vi "PickBall.vi"() -> ()   [LabVIEW 2017]
panel:
  out "Servo Position  2":u8
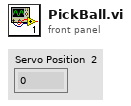
[diagram p1: front panel]
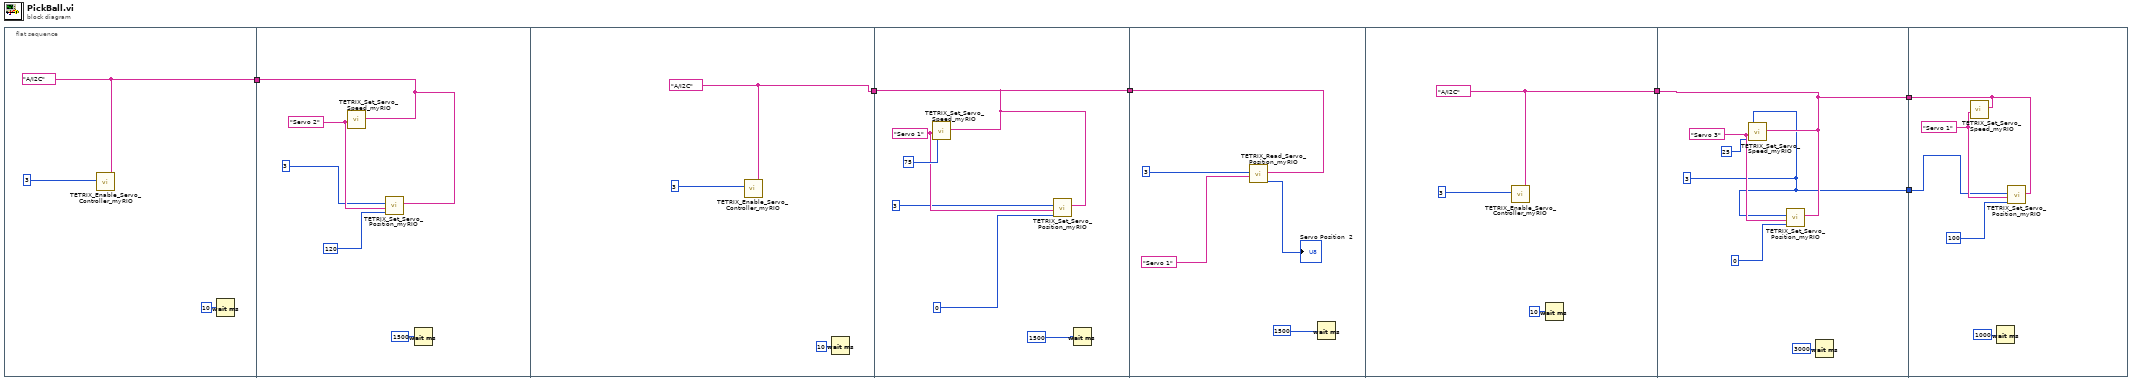
[diagram p0: block diagram]
diagram:
  n1 = flat-sequence {
    tunnel: [w8] -> w5
    tunnel: w5 -> [w10]
    tunnel: [w15] -> w3
    tunnel: [w18] -> w6
    tunnel: w3 -> [w18]
    tunnel: w6 -> [w27]
    tunnel: [w30] -> w4
    tunnel: w4 -> [w34]
    tunnel: [w33] -> w2
    tunnel: [w34] -> w1
    tunnel: w2 -> [w39]
    tunnel: w1 -> [w38]
    frame #0 {
      w8 = tag "A/I2C" ("myRIO MXP Port A/B")
      n2 = call <vilib>:"TETRIX_Enable_Servo_Controller_myRIO.vi"("myRIO MXP Port A/B"=w8, "Controller ID#  (I2C Address)"=u8 3) -> ()  [unwired: 5 in, 1 out]
      n3 = Wait (ms)(milliseconds to wait=u32 10) -> ()  [unwired: 1 out]
    }
    frame #1 {
      w14 = "Servo 2" ("Select Channel")
      n4 = call <vilib>:"TETRIX_Set_Servo_Speed_myRIO.vi"("myRIO MXP Port A/B"=w10, "Select Channel"=w14) -> ()  [unwired: 5 in, 1 out]
      n5 = call <vilib>:"TETRIX_Set_Servo_Position_myRIO.vi"("myRIO MXP Port A/B"=w10, "Set Servo Position (0 - 180 degrees)"=u8 120, "Select Channel"=w14, "Controller ID#  (I2C Address)"=u8 3) -> ()  [unwired: 3 in, 1 out]
      n6 = Wait (ms)(milliseconds to wait=u32 1500) -> ()  [unwired: 1 out]
    }
    frame #2 {
      w15 = tag "A/I2C" ("myRIO MXP Port A/B")
      n7 = call <vilib>:"TETRIX_Enable_Servo_Controller_myRIO.vi"("myRIO MXP Port A/B"=w15, "Controller ID#  (I2C Address)"=u8 3) -> ()  [unwired: 5 in, 1 out]
      n8 = Wait (ms)(milliseconds to wait=u32 10) -> ()  [unwired: 1 out]
    }
    frame #3 {
      w22 = "Servo 1" ("Select Channel")
      n9 = call <vilib>:"TETRIX_Set_Servo_Speed_myRIO.vi"("myRIO MXP Port A/B"=w18, "Set Servo Speed (0 - 100 percent)"=u8 75, "Select Channel"=w22) -> ()  [unwired: 4 in, 1 out]
      n10 = call <vilib>:"TETRIX_Set_Servo_Position_myRIO.vi"("myRIO MXP Port A/B"=w18, "Set Servo Position (0 - 180 degrees)"=u8 0, "Select Channel"=w22, "Controller ID#  (I2C Address)"=u8 3) -> ()  [unwired: 3 in, 1 out]
      n11 = Wait (ms)(milliseconds to wait=u32 1500 ("millisecond timer value")) -> ()  [unwired: 1 out]
    }
    frame #4 {
      n12 = call <vilib>:"TETRIX_Read_Servo_Position_myRIO.vi"("myRIO MXP Port A/B"=w27, "Select Channel"="Servo 1", "Controller ID#  (I2C Address)"=u8 3) -> ("Servo Position"=→"Servo Position  2":u8)  [unwired: 3 in, 1 out]
      n13 = Wait (ms)(milliseconds to wait=u32 1500 ("millisecond timer value")) -> ()  [unwired: 1 out]
    }
    frame #5 {
      w30 = tag "A/I2C" ("myRIO MXP Port A/B")
      n14 = call <vilib>:"TETRIX_Enable_Servo_Controller_myRIO.vi"("myRIO MXP Port A/B"=w30, "Controller ID#  (I2C Address)"=u8 3) -> ()  [unwired: 5 in, 1 out]
      n15 = Wait (ms)(milliseconds to wait=u32 10) -> ()  [unwired: 1 out]
    }
    frame #6 {
      w33 = u8 3 ("Controller ID#  (I2C Address)")
      w37 = "Servo 3" ("Select Channel")
      n16 = call <vilib>:"TETRIX_Set_Servo_Speed_myRIO.vi"("myRIO MXP Port A/B"=w34, "Set Servo Speed (0 - 100 percent)"=u8 25, "Select Channel"=w37, "Controller ID#  (I2C Address)"=w33) -> ()  [unwired: 3 in, 1 out]
      n17 = call <vilib>:"TETRIX_Set_Servo_Position_myRIO.vi"("myRIO MXP Port A/B"=w34, "Set Servo Position (0 - 180 degrees)"=u8 0, "Select Channel"=w37, "Controller ID#  (I2C Address)"=w33) -> ()  [unwired: 3 in, 1 out]
      n18 = Wait (ms)(milliseconds to wait=u32 3000) -> ()  [unwired: 1 out]
    }
    frame #7 {
      w41 = "Servo 1" ("Select Channel")
      n19 = call <vilib>:"TETRIX_Set_Servo_Speed_myRIO.vi"("myRIO MXP Port A/B"=w38, "Select Channel"=w41) -> ()  [unwired: 5 in, 1 out]
      n20 = Wait (ms)(milliseconds to wait=u32 1000) -> ()  [unwired: 1 out]
      n21 = call <vilib>:"TETRIX_Set_Servo_Position_myRIO.vi"("myRIO MXP Port A/B"=w38, "Set Servo Position (0 - 180 degrees)"=u8 100, "Select Channel"=w41, "Controller ID#  (I2C Address)"=w39) -> ()  [unwired: 3 in, 1 out]
    }
  }
